vi "Generate Intermediate Bezier.vi"(0 "Curve 1":T1[](array[typedef]), 1 "N":i32, 3 "Curve 2":T1[](array[typedef]), 4 "I":i32) -> (6 "Curve I":T1[](array[typedef]))   [LabVIEW 2019, in "Tool Funnel.lvclass"]
uses:
  Tool Funnel.lvclass
  Parse/PathCommands/Point.ctl
  Parse/PathCommands/PathCommands.lvclass
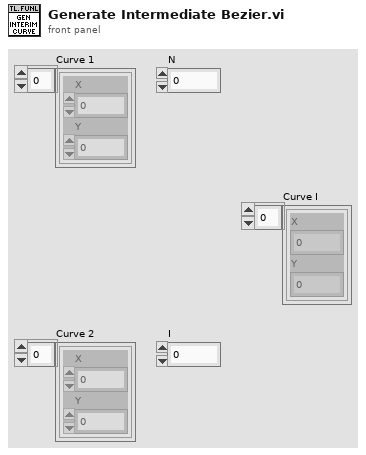
[diagram p1: front panel]
types:
  T1 = typedef "PathCommands.lvclass/Point.ctl" = cluster{"X":dbl, "Y":dbl}
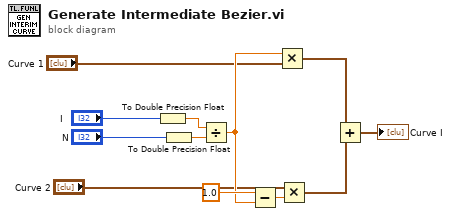
[diagram p0: block diagram]
diagram:
  n1 = To Double Precision Float(number="I") -> (double precision float=w3:dbl)
  n2 = To Double Precision Float(number="N") -> (double precision float=w2:dbl)
  n3 = Divide(x=w3, y=w2) -> (x/y=w11:dbl)
  n4 = Subtract(x=1.0, y=w11) -> (x-y=w10:dbl)
  n5 = Multiply(x=w11, y="Curve 1") -> (x*y=w9:T1[])
  n6 = Multiply(x="Curve 2", y=w10) -> (x*y=w8:T1[])
  n7 = Add(x=w9, y=w8) -> (x+y=→"Curve I":T1[])
